vi "Start Octave.vi"(8 "error in (no error)":errorcluster, 10 "Octave paths":T1, 11 "GOLPI ref. in":T2) -> (0 "error out":errorcluster, 3 "GOLPI ref. out":T2)   [LabVIEW 2020]
doc: "Starts GNU Octave if not running."
uses:
  external libraries/GOLPI 0.7.3.1 source distribution LV 20.0 32 bit/GOLPI library.lvlib
  external libraries/GOLPI 0.7.3.1 source distribution LV 20.0 32 bit/Pipe Handle.ctl
  external libraries/GOLPI 0.7.3.1 source distribution LV 20.0 32 bit/LV Process library.lvlib
  external libraries/GOLPI 0.7.3.1 source distribution LV 20.0 32 bit/GOLPI reference Type Def.ctl
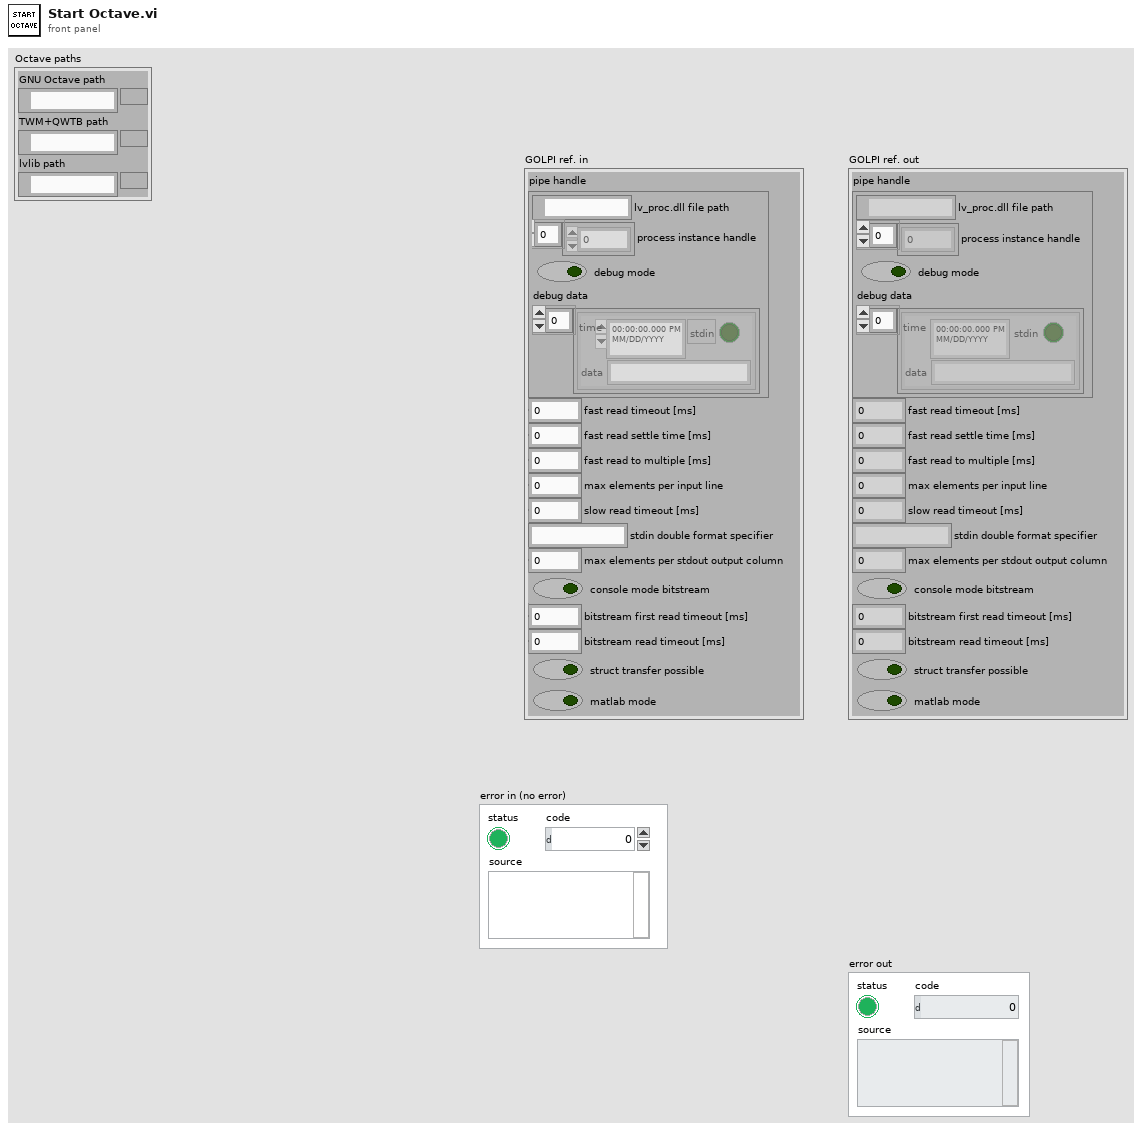
[diagram p1: front panel]
types:
  T1 = cluster{"GNU Octave path":path, "TWM+QWTB path":path, "lvlib path":path}
  T2 = typedef "GOLPI library.lvlib/GOLPI reference Type Def.ctl" = cluster{"pipe handle":T3, "fast read timeout [ms]":u32, "fast read settle time [ms]":u32, "fast read to multiple [ms]":u32, "max elements per input line":u32, "slow read timeout [ms]":u32, "stdin double format specifier":string, "max elements per stdout output column":u32, "console mode bitstream":bool, "bitstream first read timeout [ms]":u32, "bitstream read timeout [ms]":u32, "struct transfer possible":bool, "matlab mode":bool}
  T3 = typedef "LV Process library.lvlib/Pipe Handle.ctl" = cluster{"lv_proc.dll file path":path, "process instance handle":u32[], "debug mode":bool, "debug data":cluster{"time":timestamp, "stdin":bool, "data":string}[]}
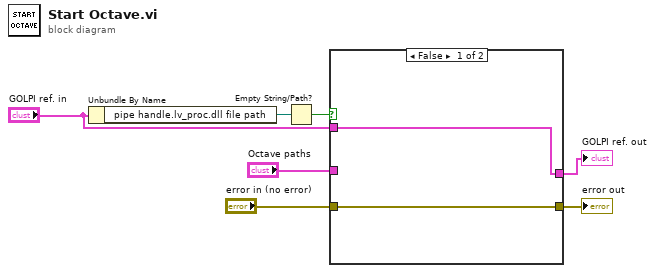
[diagram p0: block diagram]
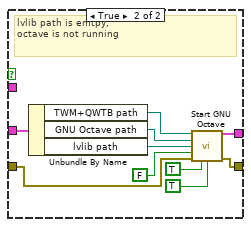
[diagram p2: hidden frame]
diagram:
  n1 = Unbundle By Name("GOLPI ref. in") -> ("pipe handle.lv_proc.dll file path"=w3:path)
  n2 = Empty String/Path?(string/path=w3) -> (empty?=w2:bool)
  n3 = case shown="False" w2 {
    tunnel: "error in (no error)" -> [w8 w19]
    tunnel: [w8 w17] -> w5
    tunnel: [w9 w16] -> w6
    tunnel: "GOLPI ref. in" -> [w9 _]
    tunnel: "Octave paths" -> [_ w14]
    frame False {
    }
    frame True {
      # "lvlib path is emtpy,\noctave is not running"
      n4 = Unbundle By Name(w14) -> ("TWM+QWTB path"=w13:path, "GNU Octave path"=w11:path, "lvlib path"=w12:path)
      n5 = call "Start GNU Octave.vi"("working dir (user home)"=w13, "octave binary file or dir (autofind)"=w11, "path to lv_proc.dll (.)"=w12, "hide debug console (T)"=FALSE, "error in"=w19, "wait for full start (T)"=TRUE, "disable history (T)"=TRUE) -> ("GOLPI ref. out"=w16:T2, "error out"=w17:errorcluster)  [unwired: 5 in, 2 out]
    }
  }
  "GOLPI ref. out" <- w6
  "error out" <- w5
